vi "AnalyzeLowRateData.vi"(8 "error in (no error)":errorcluster, 9 "data in":T13, 11 "Analysis Configuration In":T1) -> (0 "error out":errorcluster, 1 "data out":T13, 3 "Analysis Configuration Out":T1)   [LabVIEW 2017, in "McsaAnalysisLowRate.lvlib"]
uses:
  <vilib>/addons/InsightCM/Devices/Shared/Mcsa/McsaAnalysisLowRate/McsaAnalysisLowRate.lvlib
  <vilib>/addons/InsightCM/Devices/Shared/Common/DataFlow/controls/Data.ctl
  <vilib>/addons/InsightCM/Utilities/DataAccessors/controls/wfmSGL_DVR.ctl
  <vilib>/addons/PointValueMap/controls/PointMap.ctl
  <vilib>/addons/InsightCM/Devices/Shared/Common/DataFlow/controls/Type.ctl
  <vilib>/addons/InsightCM/Devices/Shared/Mcsa/McsaAnalysisLowRate/controls/Config.ctl
  <vilib>/addons/InsightCM/Devices/Shared/Mcsa/McsaAnalysisLowRate/controls/Group.ctl
  <vilib>/addons/InsightCM/Utilities/Analysis/MCSA/controls/McsaChannel.ctl
  <vilib>/addons/InsightCM/Utilities/Analysis/Shared/controls/Feature.ctl
  <vilib>/addons/InsightCM/Utilities/Analysis/Shared/controls/AmplitudeScale.ctl
  <vilib>/addons/InsightCM/MessageBus/Base/controls/KeyValuePair.ctl
  <vilib>/addons/InsightCM/Utilities/Analysis/MCSA/controls/McsaChannelPhasor.ctl
  <vilib>/addons/InsightCM/Utilities/Analysis/MCSA/controls/McsaMotor.ctl
  <vilib>/addons/InsightCM/Utilities/Analysis/MCSA/controls/MotorCalculationCache.ctl
  <vilib>/addons/Electrical Power/Basic/Measurement/subVIs/basic_Power Value.ctl
  <vilib>/addons/InsightCM/Utilities/Analysis/MCSA/controls/TorqueLoadEfficiency.ctl
  <vilib>/addons/InsightCM/Utilities/Analysis/MCSA/controls/WorkingCurrent.ctl
  <vilib>/addons/InsightCM/Devices/Shared/Mcsa/McsaResourceSchedulerLR/McsaResourceSchedulerLR.lvlib
  <vilib>/addons/PointValueMap/PointValueMap.lvlib
  <vilib>/addons/InsightCM/Devices/Shared/Common/DataFlow/DataFlow.lvlib
  <vilib>/addons/InsightCM/Utilities/Analysis/Shared/AnalysisHelper.lvlib
  <vilib>/addons/InsightCM/Utilities/Analysis/MCSA/McsaAnalysisFunctions.lvlib
  <vilib>/addons/Electrical Power/Basic/NI_EP_Basic.lvlib
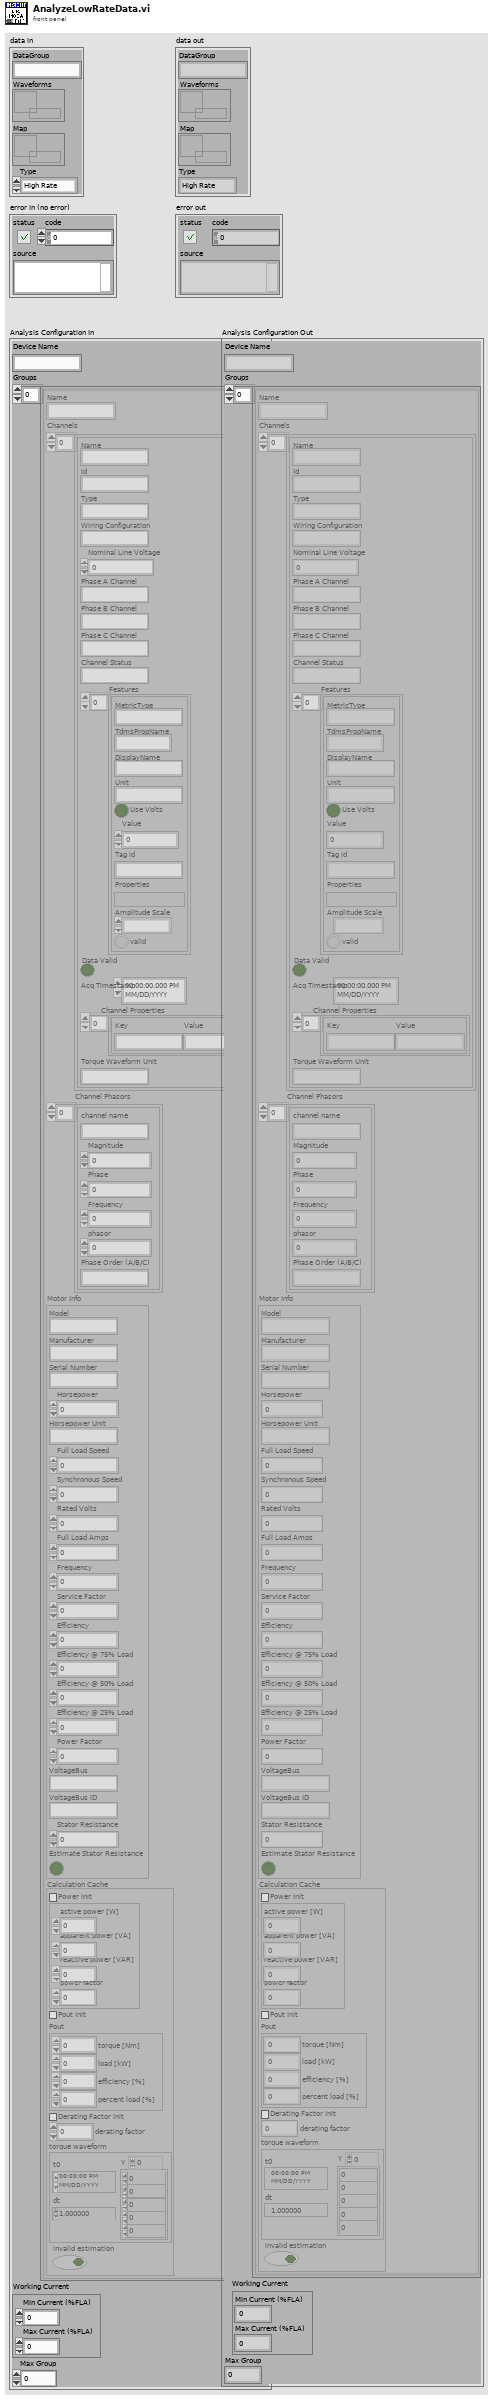
[diagram p1: front panel]
types:
  T1 = typedef "McsaAnalysisLowRate.lvlib/Config.ctl" = cluster{"Device Name":string, "Groups":T2[], "Working Current":T12, "Max Group":i32}
  T2 = typedef "McsaAnalysisLowRate.lvlib/Group.ctl" = cluster{"Name":string, "Channels":T3[], "Channel Phasors":T7[], "Motor Info":T8, "Calculation Cache":T9}
  T3 = typedef "McsaAnalysisFunctions.lvlib/McsaChannel.ctl" = cluster{"Name":string, "Id":string, "Type":string, "Wiring Configuration":string, "Nominal Line Voltage":dbl, "Phase A Channel":string, "Phase B Channel":string, "Phase C Channel":string, "Channel Status":string, "Features":T4[], "Data Valid":bool, "Acq Timestamp":timestamp, "Channel Properties":T6[], "Torque Waveform Unit":string}
  T4 = typedef "AnalysisHelper.lvlib/Feature.ctl" = cluster{"MetricType":string, "TdmsPropName":string, "DisplayName":string, "Unit":string, "Use Volts":bool, "Value":dbl, "Tag Id":string, "Properties":variant, "Amplitude Scale":T5, "valid":bool}
  T5 = typedef "AnalysisHelper.lvlib/AmplitudeScale.ctl" = enum16{"rms", "peak", "pk-pk"}
  T6 = typedef "KeyValuePair.ctl" = cluster{"Key":string, "Value":string}
  T7 = typedef "McsaAnalysisFunctions.lvlib/McsaChannelPhasor.ctl" = cluster{"channel name":string, "Magnitude":dbl, "Phase":dbl, "Frequency":dbl, "phasor":cdb, "Phase Order (A/B/C)":string}
  T8 = typedef "McsaAnalysisFunctions.lvlib/McsaMotor.ctl" = cluster{"Model":string, "Manufacturer":string, "Serial Number":string, "Horsepower":dbl, "Horsepower Unit":string, "Full Load Speed":dbl, "Synchronous Speed":dbl, "Rated Volts":dbl, "Full Load Amps":dbl, "Frequency":dbl, "Service Factor":dbl, "Efficiency":dbl, "Efficiency @ 75% Load":dbl, "Efficiency @ 50% Load":dbl, "Efficiency @ 25% Load":dbl, "Power Factor":dbl, "VoltageBus":string, "VoltageBus ID":string, "Stator Resistance":dbl, "Estimate Stator Resistance":bool}
  T9 = typedef "McsaAnalysisFunctions.lvlib/MotorCalculationCache.ctl" = cluster{"Power Init":bool, "power value":T10, "Pout Init":bool, "Pout":T11, "Derating Factor Init":bool, "derating factor":sgl, "torque waveform":waveform(dbl), "invalid estimation":bool}
  T10 = typedef "NI_EP_Basic.lvlib/basic_Power Value.ctl" = cluster{"active power [W]":dbl, "apparent power [VA]":dbl, "reactive power [VAR]":dbl, "power factor":dbl}
  T11 = typedef "McsaAnalysisFunctions.lvlib/TorqueLoadEfficiency.ctl" = cluster{"torque [Nm]":dbl, "load [kW]":dbl, "efficiency [%]":dbl, "percent load [%]":dbl}
  T12 = typedef "McsaAnalysisFunctions.lvlib/WorkingCurrent.ctl" = cluster{"Min Current (%FLA)":dbl, "Max Current (%FLA)":dbl}
  T13 = typedef "DataFlow.lvlib/Data.ctl" = cluster{"DataGroup":string, "Waveforms":T14, "Map":T15, "Type":T16}
  T14 = typedef "wfmSGL_DVR.ctl" = refnum<data-value>
  T15 = typedef "PointValueMap.lvlib/PointMap.ctl" = refnum<data-value>
  T16 = typedef "DataFlow.lvlib/Type.ctl" = enum16{"High Rate", "Low Rate", "Burst Mode"}
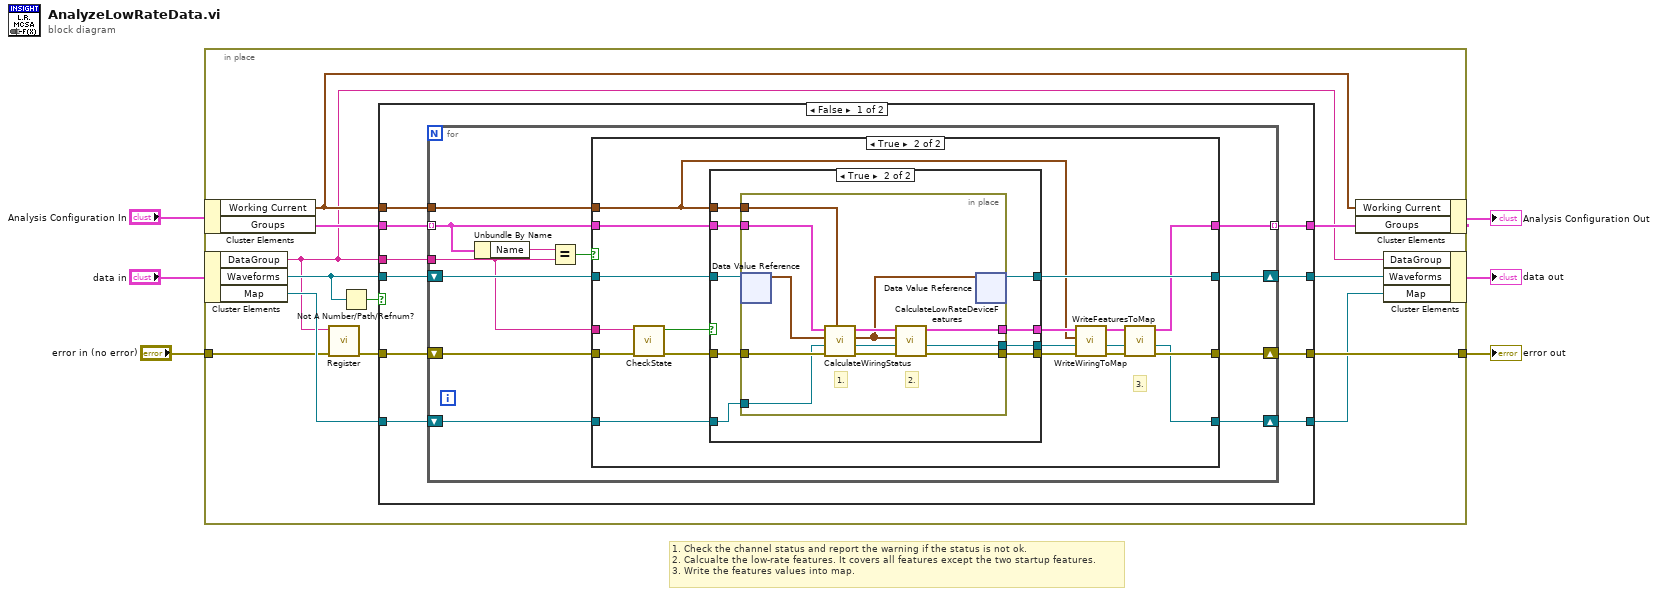
[diagram p0: block diagram]
diagram:
  # "1. Check the channel status and report the warning if the status is not ok.\n2. Calcualte the low-rate features. It covers all features except the two startup features.\n3. Write the features values into map."
  n1 = in-place {
    in-place-border: [w18] -> w3
    in-place-border: "error in (no error)" -> [w9]
    n2 = in-place-cluster #1("Analysis Configuration In") -> ("Working Current"=w10:T12, "Groups"=w17:T2[])
    n3 = in-place-cluster #2("data in") -> ("DataGroup"=w7:string, "Waveforms"=w12:T14, "Map"=w15:T15)
    n4 = call <vilib>:"Register.vi"("error in (no error)"=w9, "name"=w7) -> ("error out"=w8:errorcluster)  [unwired: 9 in]
    n5 = Not A Number/Path/Refnum?(number/path/refnum=w12) -> (NaN/Path/Refnum?=w11:bool)
    n6 = case shown="False" w11 {
      tunnel: [w28 w89] -> w18
      tunnel: w17 -> [w27 w91]
      tunnel: [w26 w91] -> w16
      tunnel: w8 -> [w25 w89]
      tunnel: w15 -> [w24 w88]
      tunnel: [w23 w90] -> w14
      tunnel: w7 -> [w22 _]
      tunnel: [w21 w88] -> w13
      tunnel: w12 -> [w20 w90]
      tunnel: w10 -> [w19 _]
      frame False {
        n7 = for {
          tunnel: w22 -> [w29]
          shift-right: [w40] -> w28
          shift-left: w25 -> [w37]
          tunnel: w27 -> [w34] mode=indexing
          tunnel: [w33] -> w26 mode=indexing
          shift-right: [w32] -> w23
          shift-left: w20 -> [w39]
          shift-right: [w31] -> w21
          shift-left: w24 -> [w38]
          tunnel: w19 -> [w30]
          n8 = Unbundle By Name(w34) -> ("Name"=w36:string)
          n9 = Equal?(x=w36, y=w29) -> (x = y?=w35:bool)
          n10 = case shown="True" w35 {
            tunnel: [w43 w54] -> w40
            tunnel: w39 -> [w42 w62]
            tunnel: w38 -> [w41 w61]
            tunnel: w37 -> [w43 w58]
            tunnel: w34 -> [w44 w60]
            tunnel: [w44 w52] -> w33
            tunnel: [w42 w59] -> w32
            tunnel: [w41 w53] -> w31
            tunnel: w30 -> [_ w45]
            tunnel: w29 -> [_ w55]
            frame False {
            }
            frame True {
              # "3."
              n11 = call <vilib>:"CheckState.vi"("error in (no error)"=w58, "name"=w55) -> ("error out"=w57:errorcluster, "active"=w56:bool)  [unwired: 8 in]
              n12 = case shown="True" w56 {
                tunnel: [w65 w68] -> w46
                tunnel: w62 -> [w66 w75]
                tunnel: w61 -> [w63 w74]
                tunnel: w57 -> [w65 w73]
                tunnel: w60 -> [w64 w72]
                tunnel: [w66 w71] -> w59
                tunnel: w45 -> [_ w70]
                tunnel: [w64 w69] -> w51
                tunnel: [w63 w67] -> w47
                frame False {
                }
                frame True {
                  n13 = in-place {
                    in-place-border: w73 -> [w87]
                    in-place-border: w74 -> [w86]
                    in-place-border: w72 -> [w83]
                    in-place-border: w70 -> [w76]
                    in-place-border: [w79] -> w69
                    in-place-border: [w78] -> w68
                    in-place-border: [w77] -> w67
                    # "2."
                    # "1."
                    n14 = in-place-dvr #3(w75) -> (w84:waveform(sgl)[])  [unwired: 1 out]
                    n15 = call <vilib>:"CalculateWiringStatus.vi"("Working Current"=w76, "error in (no error)"=w87, "map in"=w86, "Waveforms"=w84, "Group in"=w83) -> ("error out"=w85:errorcluster, "Map out"=w81:T15, "Waveforms Out"=w80:waveform(sgl)[], "Group out"=w82:T2)  [unwired: 3 in]
                    n16 = call <vilib>:"CalculateLowRateDeviceFeatures.vi"("error in (no error)"=w85, "data flow map in"=w81, "Waveforms"=w80, "Group in"=w82) -> ("error out"=w78:errorcluster, "data flow map out"=w77:T15, "Group out"=w79:T2)  [unwired: 5 in]
                    n17 = in-place-dvr #3(w80) -> (w71:T14)  [unwired: 1 out]
                  }
                }
              }
              n18 = call <vilib>:"WriteWiringToMap.vi"("error in (no error)"=w46, "Map in"=w47, "Working Current"=w45, "Group"=w51) -> ("error out"=w49:errorcluster, "Map out"=w48:T15, "Group out"=w50:T2)  [unwired: 5 in]
              n19 = call <vilib>:"WriteFeaturesToMap.vi"("error in (no error)"=w49, "Map in"=w48, "Group"=w50) -> ("error out"=w54:errorcluster, "Map out"=w53:T15, "Group out"=w52:T2)  [unwired: 6 in]
            }
          }
        }
      }
      frame True {
      }
    }
    n20 = in-place-cluster #1("Working Current"=w10, "Groups"=w16) -> (→"Analysis Configuration Out":T1)
    n21 = in-place-cluster #2("DataGroup"=w7, "Waveforms"=w14, "Map"=w13) -> (→"data out":T13)
  }
  "error out" <- w3
